vi "test-rotation2d.vi"() -> ()   [LabVIEW 2019]
uses:
  <vilib>/Rock Robotics/WPI/ThirdParty/JAS_Junk/TrajLib/Util_CalcDist.vi
  <vilib>/Rock Robotics/WPI/ThirdParty/JAS_Junk/TrajLib/Rotation_UnaryMinus.vi
  <vilib>/Rock Robotics/WPI/ThirdParty/JAS_Junk/TrajLib/Rotation_CreateXY.vi
  <vilib>/Rock Robotics/WPI/ThirdParty/JAS_Junk/TrajLib/Trajectory_Library.lvlib
panel:
  out "T7 - True":bool
  out "T4 -- X -- 0":dbl
  out "T3 -- X -- 0":dbl
  out "T2 -- y -- 0":dbl
  out "T2 -- X -- 0":dbl
  out "T6 - False":bool
  out "T5 - True":bool
  out "T1 -- y -- 0":dbl
  out "T1 -- X -- 0":dbl
  out "T0 -- y -- 0":dbl
  out "T0 -- X -- 0":dbl
  # "Rotation2D Test"
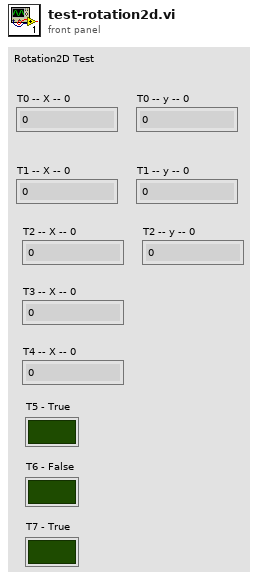
[diagram p1: front panel]
types:
  T1 = typedef "Trajectory_Library.lvlib/ROTATION2D.ctl" = cluster{"VALUE":dbl, "COS":dbl, "SIN":dbl}
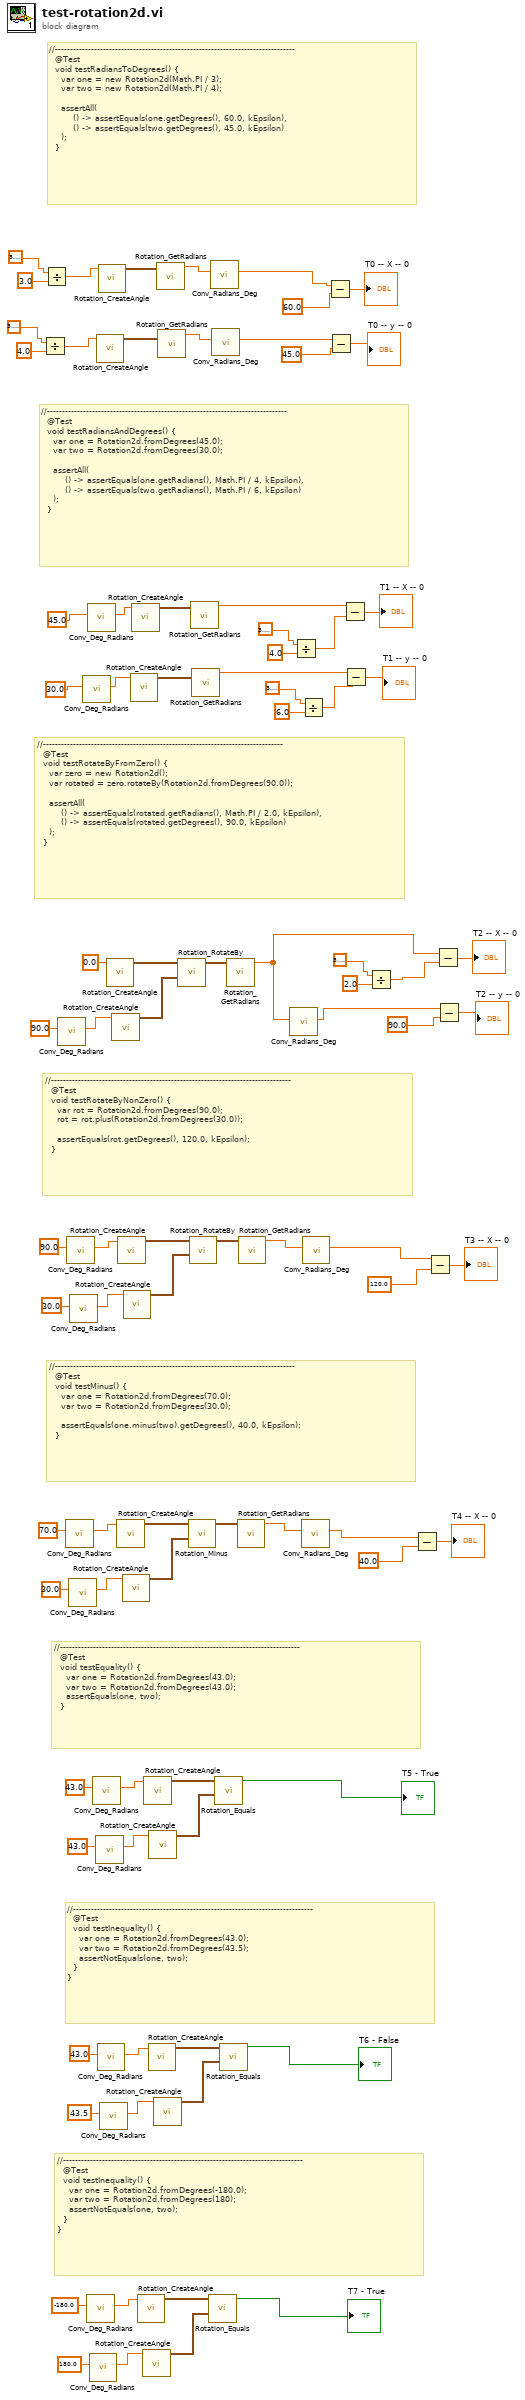
[diagram p0: block diagram]
diagram:
  # "//--------------------------------------------------------------------------------\n  @Test\n  void testInequality() {\n    var one = Rotation2d.fromDegrees(-180.0);\n    var two = Rotation2d.fromDegrees(180);\n    assertNotEquals(one, two);\n  }\n}"
  # "//--------------------------------------------------------------------------------\n  @Test\n  void testInequality() {\n    var one = Rotation2d.fromDegrees(43.0);\n    var two = Rotation2d.fromDegrees(43.5);\n    assertNotEquals(one, two);\n  }\n}"
  # "//--------------------------------------------------------------------------------\n  @Test\n  void testMinus() {\n    var one = Rotation2d.fromDegrees(70.0);\n    var two = Rotation2d.fromDegrees(30.0);\n\n    assertEquals(one.minus(two).getDegrees(), 40.0, kEpsilon);\n  }"
  # "//--------------------------------------------------------------------------------\n  @Test\n  void testRotateByNonZero() {\n    var rot = Rotation2d.fromDegrees(90.0);\n    rot = rot.plus(Rotation2d.fromDegrees(30.0));\n\n    assertEquals(rot.getDegrees(), 120.0, kEpsilon);\n  }"
  # "//--------------------------------------------------------------------------------\n  @Test\n  void testRotateByFromZero() {\n    var zero = new Rotation2d();\n    var rotated = zero.rotateBy(Rotation2d.fromDegrees(90.0));\n\n    assertAll(\n        () -> assertEquals(rotated.getRadians(), Math.PI / 2.0, kEpsilon),\n        () -> assertEquals(rotated.getDegrees(), 90.0, kEpsilon)\n    );\n  }"
  # "//--------------------------------------------------------------------------------\n  @Test\n  void testEquality() {\n    var one = Rotation2d.fromDegrees(43.0);\n    var two = Rotation2d.fromDegrees(43.0);\n    assertEquals(one, two);\n  }"
  # "//--------------------------------------------------------------------------------\n  @Test\n  void testRadiansAndDegrees() {\n    var one = Rotation2d.fromDegrees(45.0);\n    var two = Rotation2d.fromDegrees(30.0);\n\n    assertAll(\n        () -> assertEquals(one.getRadians(), Math.PI / 4, kEpsilon),\n        () -> assertEquals(two.getRadians(), Math.PI / 6, kEpsilon)\n    );\n  }"
  # "//--------------------------------------------------------------------------------\n  @Test\n  void testRadiansToDegrees() {\n    var one = new Rotation2d(Math.PI / 3);\n    var two = new Rotation2d(Math.PI / 4);\n\n    assertAll(\n        () -> assertEquals(one.getDegrees(), 60.0, kEpsilon),\n        () -> assertEquals(two.getDegrees(), 45.0, kEpsilon)\n    );\n  }"
  n1 = Divide(x=3.141592653589793, y=4.0) -> (x/y=w69:dbl)
  n2 = Divide(x=3.141592653589793, y=3.0) -> (x/y=w72:dbl)
  n3 = call <vilib>:"Conv_Deg_Radians.vi"("Degress"=90.0) -> ("Radians"=w80:dbl)  [unwired: 10 in]
  n4 = call <vilib>:"Conv_Deg_Radians.vi"("Degress"=70.0) -> ("Radians"=w23:dbl)  [unwired: 10 in]
  n5 = call <vilib>:"Conv_Deg_Radians.vi"("Degress"=90.0) -> ("Radians"=w32:dbl)  [unwired: 10 in]
  n6 = call <vilib>:"Conv_Deg_Radians.vi"("Degress"=30.0) -> ("Radians"=w30:dbl)  [unwired: 10 in]
  n7 = call <vilib>:"Conv_Deg_Radians.vi"("Degress"=30.0) -> ("Radians"=w39:dbl)  [unwired: 10 in]
  n8 = call <vilib>:"Conv_Deg_Radians.vi"("Degress"=30.0 ("y")) -> ("Radians"=w54:dbl)  [unwired: 10 in]
  n9 = call <vilib>:"Conv_Deg_Radians.vi"("Degress"=-180.0) -> ("Radians"=w2:dbl)  [unwired: 10 in]
  n10 = call <vilib>:"Conv_Deg_Radians.vi"("Degress"=45.0 ("y")) -> ("Radians"=w53:dbl)  [unwired: 10 in]
  n11 = call <vilib>:"Conv_Deg_Radians.vi"("Degress"=180.0) -> ("Radians"=w7:dbl)  [unwired: 10 in]
  n12 = call <vilib>:"Conv_Deg_Radians.vi"("Degress"=43.0) -> ("Radians"=w16:dbl)  [unwired: 10 in]
  n13 = call <vilib>:"Conv_Deg_Radians.vi"("Degress"=43.0) -> ("Radians"=w21:dbl)  [unwired: 10 in]
  n14 = call <vilib>:"Rotation_CreateAngle.vi"("Angle"=w69) -> ("ROTATION"=w65:T1)  [unwired: 10 in]
  n15 = call <vilib>:"Conv_Deg_Radians.vi"("Degress"=43.0) -> ("Radians"=w9:dbl)  [unwired: 10 in]
  n16 = call <vilib>:"Rotation_CreateAngle.vi"("Angle"=w72) -> ("ROTATION"=w68:T1)  [unwired: 10 in]
  n17 = call <vilib>:"Conv_Deg_Radians.vi"("Degress"=43.5) -> ("Radians"=w14:dbl)  [unwired: 10 in]
  n18 = call <vilib>:"Rotation_CreateAngle.vi"("Angle"=0.0) -> ("ROTATION"=w47:T1)  [unwired: 10 in]
  n19 = call <vilib>:"Rotation_CreateAngle.vi"("Angle"=w80) -> ("ROTATION"=w46:T1)  [unwired: 10 in]
  n20 = call <vilib>:"Rotation_CreateAngle.vi"("Angle"=w23) -> ("ROTATION"=w28:T1)  [unwired: 10 in]
  n21 = call <vilib>:"Rotation_CreateAngle.vi"("Angle"=w32) -> ("ROTATION"=w37:T1)  [unwired: 10 in]
  n22 = call <vilib>:"Rotation_CreateAngle.vi"("Angle"=w30) -> ("ROTATION"=w27:T1)  [unwired: 10 in]
  n23 = call <vilib>:"Rotation_CreateAngle.vi"("Angle"=w39) -> ("ROTATION"=w36:T1)  [unwired: 10 in]
  n24 = call <vilib>:"Rotation_CreateAngle.vi"("Angle"=w54) -> ("ROTATION"=w61:T1)  [unwired: 10 in]
  n25 = call <vilib>:"Rotation_CreateAngle.vi"("Angle"=w53) -> ("ROTATION"=w62:T1)  [unwired: 10 in]
  n26 = call <vilib>:"Rotation_CreateAngle.vi"("Angle"=w2) -> ("ROTATION"=w5:T1)  [unwired: 10 in]
  n27 = call <vilib>:"Rotation_CreateAngle.vi"("Angle"=w7) -> ("ROTATION"=w4:T1)  [unwired: 10 in]
  n28 = call <vilib>:"Rotation_CreateAngle.vi"("Angle"=w16) -> ("ROTATION"=w19:T1)  [unwired: 10 in]
  n29 = call <vilib>:"Rotation_CreateAngle.vi"("Angle"=w9) -> ("ROTATION"=w12:T1)  [unwired: 10 in]
  n30 = call <vilib>:"Rotation_CreateAngle.vi"("Angle"=w21) -> ("ROTATION"=w18:T1)  [unwired: 10 in]
  n31 = call <vilib>:"Rotation_CreateAngle.vi"("Angle"=w14) -> ("ROTATION"=w11:T1)  [unwired: 10 in]
  n32 = call <vilib>:"Rotation_GetRadians.vi"("in ROTATION"=w68) -> ("AngleRadians"=w67:dbl)  [unwired: 10 in]
  n33 = call <vilib>:"Rotation_GetRadians.vi"("in ROTATION"=w65) -> ("AngleRadians"=w66:dbl)  [unwired: 10 in]
  n34 = call <vilib>:"Rotation_RotateBy.vi"("other Rotation"=w46, "in ROTATION"=w47) -> ("out ROTATION"=w45:T1)  [unwired: 9 in]
  n35 = call <vilib>:"Rotation_Minus.vi"("other ROTATION"=w27, "in ROTATION"=w28) -> ("out ROTATION"=w26:T1)  [unwired: 9 in]
  n36 = call <vilib>:"Rotation_RotateBy.vi"("other Rotation"=w36, "in ROTATION"=w37) -> ("out ROTATION"=w35:T1)  [unwired: 9 in]
  n37 = call <vilib>:"Rotation_GetRadians.vi"("in ROTATION"=w62) -> ("AngleRadians"=w50:dbl)  [unwired: 10 in]
  n38 = call <vilib>:"Rotation_GetRadians.vi"("in ROTATION"=w61) -> ("AngleRadians"=w49:dbl)  [unwired: 10 in]
  n39 = call <vilib>:"Rotation_Equals.vi"("other ROTATION"=w4, "in ROTATION"=w5) -> ("Equals"=→"T7 - True":bool)  [unwired: 9 in]
  n40 = call <vilib>:"Conv_Radians_Deg.vi"("Radians"=w67) -> ("Degrees"=w64:dbl)  [unwired: 10 in]
  n41 = call <vilib>:"Conv_Radians_Deg.vi"("Radians"=w66) -> ("Degrees"=w63:dbl)  [unwired: 10 in]
  n42 = call <vilib>:"Rotation_Equals.vi"("other ROTATION"=w18, "in ROTATION"=w19) -> ("Equals"=→"T5 - True":bool)  [unwired: 9 in]
  n43 = call <vilib>:"Rotation_Equals.vi"("other ROTATION"=w11, "in ROTATION"=w12) -> ("Equals"=→"T6 - False":bool)  [unwired: 9 in]
  n44 = call <vilib>:"Rotation_GetRadians.vi"("in ROTATION"=w45) -> ("AngleRadians"=w41:dbl)  [unwired: 10 in]
  n45 = call <vilib>:"Rotation_GetRadians.vi"("in ROTATION"=w26) -> ("AngleRadians"=w25:dbl)  [unwired: 10 in]
  n46 = call <vilib>:"Rotation_GetRadians.vi"("in ROTATION"=w35) -> ("AngleRadians"=w34:dbl)  [unwired: 10 in]
  n47 = call <vilib>:"Conv_Radians_Deg.vi"("Radians"=w41) -> ("Degrees"=w40:dbl)  [unwired: 10 in]
  n48 = Divide(x=3.141592653589793, y=4.0) -> (x/y=w55:dbl)
  n49 = Divide(x=3.141592653589793, y=6.0) -> (x/y=w56:dbl)
  n50 = call <vilib>:"Conv_Radians_Deg.vi"("Radians"=w25) -> ("Degrees"=w22:dbl)  [unwired: 10 in]
  n51 = call <vilib>:"Conv_Radians_Deg.vi"("Radians"=w34) -> ("Degrees"=w31:dbl)  [unwired: 10 in]
  n52 = Subtract(x=w64, y=60.0) -> (x-y=→"T0 -- X -- 0":dbl)
  n53 = Subtract(x=w63, y=45.0) -> (x-y=→"T0 -- y -- 0":dbl)
  n54 = Subtract(x=w50, y=w55) -> (x-y=→"T1 -- X -- 0":dbl)
  n55 = Subtract(x=w49, y=w56) -> (x-y=→"T1 -- y -- 0":dbl)
  n56 = Divide(x=3.141592653589793, y=2.0) -> (x/y=w42:dbl)
  n57 = Subtract(x=w22, y=40.0 ("x")) -> (x-y=→"T4 -- X -- 0":dbl)
  n58 = Subtract(x=w31, y=120.0 ("x")) -> (x-y=→"T3 -- X -- 0":dbl)
  n59 = Subtract(x=w41, y=w42) -> (x-y=→"T2 -- X -- 0":dbl)
  n60 = Subtract(x=w40, y=90.0) -> (x-y=→"T2 -- y -- 0":dbl)
